vi "Load .Obj File.vi"(5 "Load Material Textures (Default: True)":bool=TRUE, 6 "Material Search Folder (Default: Empty - Use Model Path Folder)":path, 7 "Force Regenerate Normals (Defaut: False)":bool, 8 "error in (no error)":errorcluster, 11 "Object Model Path":path) -> (0 "error out":errorcluster, 3 "Objects":refnum<vi>[](array[refnum]), 4 "Bounding Box":T1)   [LabVIEW 2020, in "ar.lvlib"]
doc: "Load a .Obj 3D Model file."
uses:
  ar.lvlib
  Model Bounding Box.ctl
  common/Object Point (Float).ctl
  Vertex Descriptor.ctl
  <vilib>/Utility/miscctls.llb/LV3DPointTypeDef.ctl
  <vilib>/picture/3D Picture Control/Geometries/Create Mesh.vi
  <vilib>/picture/3D Picture Control/Object/Create Object.vi
  <vilib>/picture/3D Picture Control/Object/Create Object (drawable).vi
  <vilib>/picture/3D Picture Control/Object/Set Material.vi
  <vilib>/Utility/libraryn.llb/Get File Extension.vi
  <vilib>/picture/jpeg.llb/Read JPEG File.vi
  <vilib>/picture/3D Picture Control/Helpers/Apply Texture.vi
  <vilib>/picture/3D Picture Control/Helpers/Apply Texture (no reference).vi
  <vilib>/picture/png.llb/Read PNG File.vi
  <vilib>/picture/bmp.llb/Read BMP File.vi
  common/common.lvlib
  common/bin/gartoolkit_ar_32-1.dll
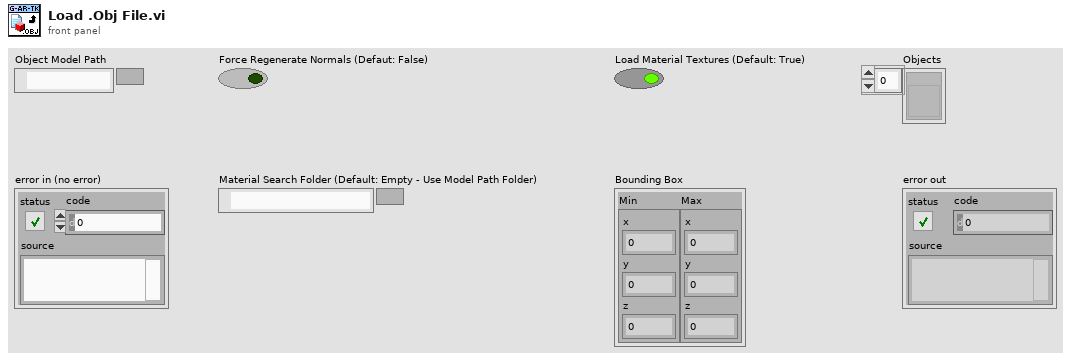
[diagram p1: front panel]
types:
  T1 = typedef "ar.lvlib/Model Bounding Box.ctl" = cluster{"Min":T2, "Max":T2}
  T2 = typedef "common.lvlib/Object Point (Float).ctl" = cluster{"x":dbl, "y":dbl, "z":dbl}
  T3 = typedef "ar.lvlib/Vertex Descriptor.ctl" = cluster{"Vertex":T4, "Normal":T4, "Colour":cluster{"R":sgl, "G":sgl, "B":sgl}, "Texture Coord":cluster{"S":sgl, "T":sgl}}
  T4 = typedef "LV3DPointTypeDef.ctl" = cluster{"X":sgl, "Y":sgl, "Z":sgl}
  T5 = cluster{"Name":string, "Shininess":sgl, "Ambient":cluster{"Red":sgl, "Green":sgl, "Blue":sgl}, "Specular":cluster{"Red":sgl, "Green":sgl, "Blue":sgl}, "Emission":cluster{"Red":sgl, "Green":sgl, "Blue":sgl}, "Diffuse":cluster{"Red":sgl, "Green":sgl, "Blue":sgl}, "texture-name":string}[]
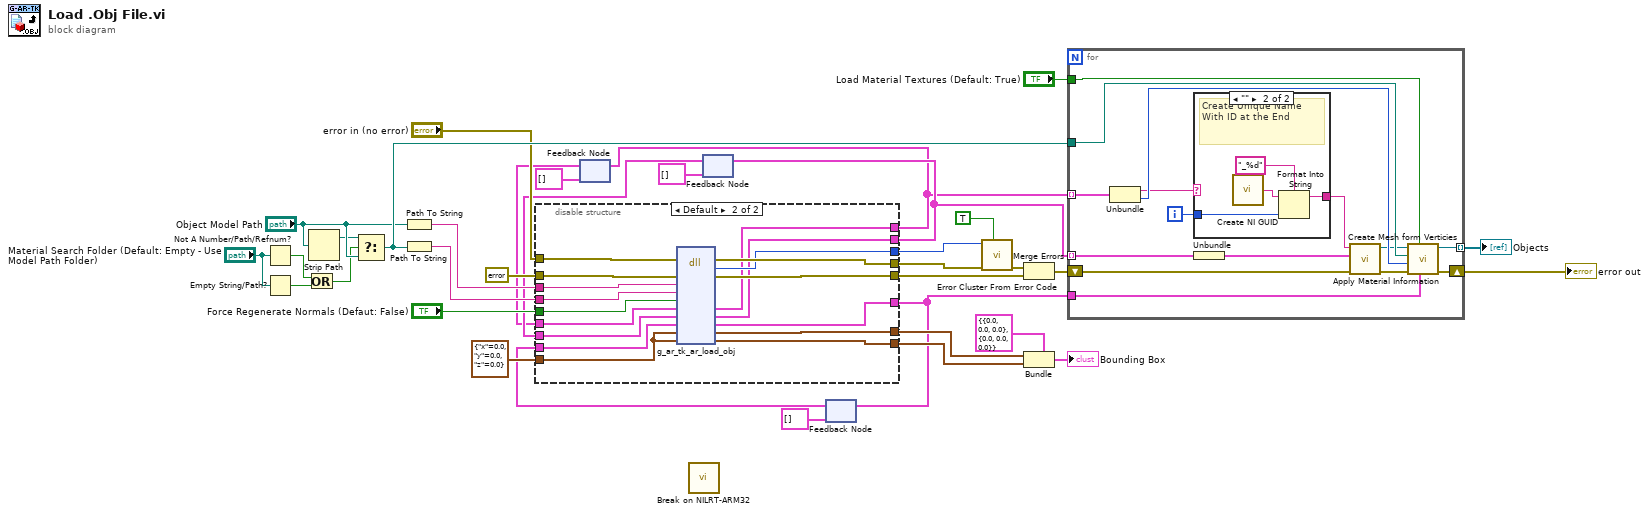
[diagram p0: block diagram]
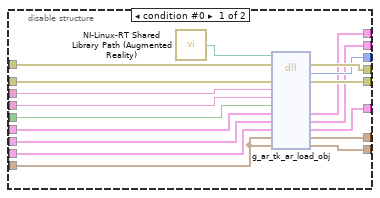
[diagram p2: hidden frame]
diagram:
  n1 = Not A Number/Path/Refnum?(number/path/refnum="Material Search Folder (Default: Empty - Use Model Path Folder)") -> (NaN/Path/Refnum?=w28:bool)
  n2 = Empty String/Path?(string/path="Material Search Folder (Default: Empty - Use Model Path Folder)") -> (empty?=w22:bool)
  n3 = Or(x=w28, y=w22) -> (x .or. y?=w23:bool)
  n4 = Strip Path(path="Object Model Path") -> (stripped path=w25:path)  [unwired: 1 out]
  n5 = Select(t=w25, s=w23, f="Object Model Path") -> (s? t:f=w27:path)
  n6 = Path To String(path="Object Model Path") -> (string=w19:string)
  n7 = Path To String(path=w27) -> (string=w18:string)
  n8 = feedback #1(cluster{"name":string, "material_id":i32}[] []) -> (w2:cluster{"name":string, "material_id":i32}[])
  n9 = call "Break on NILRT-ARM32.vi"() -> ()  [unwired: 12 in]
  n10 = feedback #2(cluster{"Verticies":T3[]}[] []) -> (w5:cluster{"Verticies":T3[]}[])
  n11 = feedback #3(T5 [] ("Materials")) -> (w8:T5)
  n12 = disable-structure shown="Default" {
    disable-tunnel: "error in (no error)" -> [w53 w70]
    disable-tunnel: errorcluster {"status"=FALSE, "code"=0, "source"=""} ("error constant") -> [w52 w69]
    disable-tunnel: w19 -> [w51 w68]
    disable-tunnel: w18 -> [w50 w67]
    disable-tunnel: "Force Regenerate Normals (Defaut: False)" -> [w49 w66]
    disable-tunnel: w2 -> [w48 w65]
    disable-tunnel: w5 -> [w47 w64]
    disable-tunnel: w8 -> [w46 w63]
    disable-tunnel: T2 {"x"=0.0, "y"=0.0, "z"=0.0} ("Object Point") -> [w45 w62]
    disable-tunnel: [w44 w61] -> w15
    disable-tunnel: [w43 w60] -> w14
    disable-tunnel: [w42 w59] -> w13
    disable-tunnel: [w41 w58] -> w3
    disable-tunnel: [w40 w57] -> w6
    disable-tunnel: [w39 w56] -> w10
    disable-tunnel: [w38 w55] -> w12
    disable-tunnel: [w37 w54] -> w11
    frame condition #0 {
      n13 = call "NI-Linux-RT Shared Library Path (Augmented Reality).vi"() -> ("Path"=w36:path)
      n14 = dll-call lib="?" fn="g_ar_tk_ar_load_obj" ("g_ar_toolkit.*.*:g_ar_tk_image_copy")(path in=w36, error in=w53, "error_cluster"=w52, "object_path"=w51, "material_path"=w50, "regen_normals"=w49, "object_array"=w48, "point_arrays"=w47, "material_array"=w46, "bbox_min"=w45, "bbox_max"=w45) -> (error out=w44:errorcluster, "mg_err_code"=w43:i32, "error_cluster"=w42:errorcluster, "object_array"=w41:cluster{"name":string, "material_id":i32}[], "point_arrays"=w40:cluster{"Verticies":T3[]}[], "material_array"=w39:T5, "bbox_min"=w38:T2, "bbox_max"=w37:T2)  [unwired: 4 in, 1 out]
    }
    frame condition #1 (active) {
      n15 = dll-call lib="C:/serenial/lib/g-augmented-reality-toolkit/LabVIEW/common/bin/gartoolkit_ar_*-1.*" fn="g_ar_tk_ar_load_obj" ("g_ar_toolkit.*.*:g_ar_tk_image_copy")(error in=w70, "error_cluster"=w69, "object_path"=w68, "material_path"=w67, "regen_normals"=w66, "object_array"=w65, "point_arrays"=w64, "material_array"=w63, "bbox_min"=w62, "bbox_max"=w62) -> (error out=w61:errorcluster, "mg_err_code"=w60:i32, "error_cluster"=w59:errorcluster, "object_array"=w58:cluster{"name":string, "material_id":i32}[], "point_arrays"=w57:cluster{"Verticies":T3[]}[], "material_array"=w56:T5, "bbox_min"=w55:T2, "bbox_max"=w54:T2)  [unwired: 5 in, 1 out]
    }
  }
  n16 = feedback-in #1(w3) -> ()
  n17 = feedback-in #2(w6) -> ()
  n18 = feedback-in #3(w10) -> ()
  n19 = call <vilib>:"Error Cluster From Error Code.vi"("show call chain? (False)"=TRUE, "error in (no error)"=w15, "error code (0)"=w14) -> ("error out"=w35:errorcluster)  [unwired: 6 in]
  n20 = Merge Errors(w35, w13) -> (w34:errorcluster)
  n21 = Bundle(cluster=T1 {"Min"={"x"=0.0, "y"=0.0, "z"=0.0}, "Max"={"x"=0.0, "y"=0.0, "z"=0.0}} ("Bounding Box"), "Min"=w12, "Max"=w11) -> (→"Bounding Box":T1)
  n22 = for {
    tunnel: w3 -> [w85] mode=indexing
    tunnel: [w84] -> w33 mode=indexing
    tunnel: w10 -> [w82]
    shift-right: [w83] -> w32
    shift-left: w34 -> [w81]
    tunnel: w27 -> [w79]
    tunnel: w6 -> [w75] mode=indexing
    tunnel: "Load Material Textures (Default: True)" -> [w71]
    i -> [w77]
    n23 = Unbundle(w85) -> ("name"=w78:string, "material_id"=w80:i32)
    n24 = case shown="\"\"" w78 {
      selector: w78 -> [w86 _]
      tunnel: w77 -> [_ w90]
      tunnel: [w86 w87] -> w76
      frame Default {
      }
      frame "" {
        # "Create Unique Name With ID at the End"
        n25 = call <vilib>:"Create NI GUID.vi"() -> ("NI GUID"=w89:string)
        n26 = Format Into String(format string="_%d", initial string=w89, w90) -> (resulting string=w87:string)  [unwired: 1 in, 1 out]
      }
    }
    n27 = Unbundle(w75) -> ("Verticies"=w74:T3[])
    n28 = call "Create Mesh form Verticies.vi"("error in (no error)"=w81, "Verticies"=w74, "Object Name"=w76) -> ("error out"=w72:errorcluster, "SceneObject out"=w73:refnum<vi>)  [unwired: 7 in]
    n29 = call "Apply Material Information.vi"("Materials"=w82, "Load Material Textures"=w71, "error in (no error)"=w72, "material_id"=w80, "Material Path"=w79, "SceneObject in"=w73) -> ("error out"=w83:errorcluster, "SceneObject out"=w84:refnum<vi>)  [unwired: 4 in]
  }
  "Objects" <- w33
  "error out" <- w32
